vi "Tusk.MessageSenderCore.vi"(5 "Priority?":bool, 7 "Timeout (ms)(-1)":i32=-1, 8 "error in (no error)":errorcluster, 10 "Message":refnum<class "Message.lvclass">, 11 "Tusk in":refnum<class "Tusk.lvclass">) -> (0 "error out":errorcluster, 1 "Timed out?":bool, 3 "Tusk out":refnum<class "Tusk.lvclass">)   [LabVIEW 2018, in "Application.lvlib" / "Tusk.lvclass"]
uses:
  Tusk.lvclass
  Message Class/Message.lvclass
  Tusk.lvclass/Tusk.ctl
  <vilib>/event_ctls.llb/usereventprio.ctl
  Exceptions Class/Exceptions.lvclass
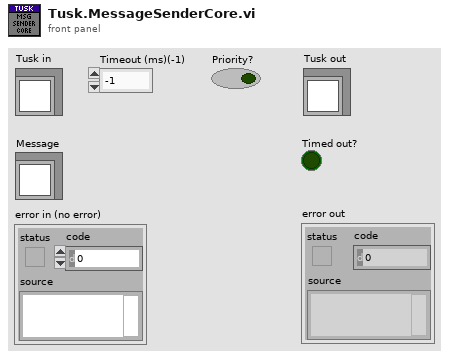
[diagram p1: front panel]
types:
  T1 = typedef "Type.ctl" = enum16{"None", "Queue", "Event", "Notifier"}
  T2 = typedef "usereventprio.ctl" = enum32{"high priority", "normal priority"}
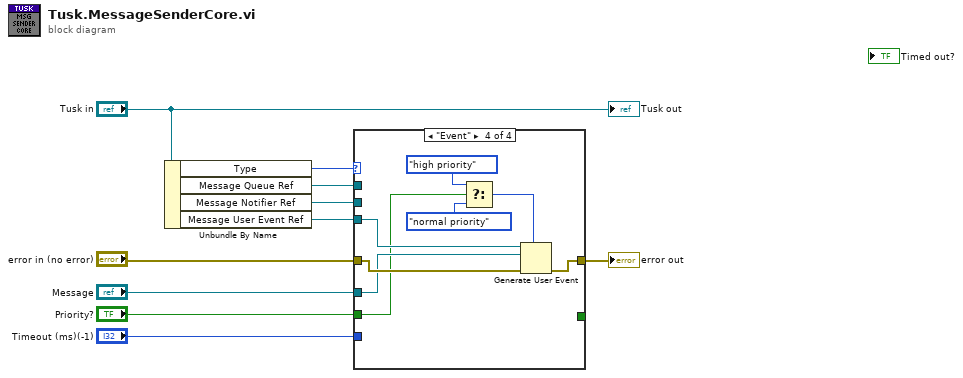
[diagram p0: block diagram]
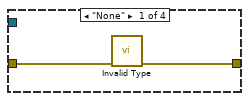
[diagram p2: hidden frame]
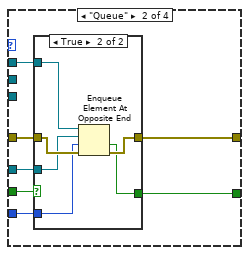
[diagram p3: hidden frame]
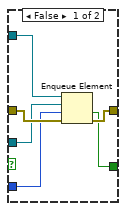
[diagram p4: hidden frame]
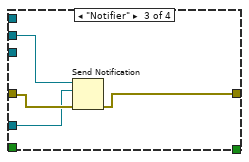
[diagram p5: hidden frame]
diagram:
  n1 = Unbundle By Name("Tusk in") -> ("Type"=w9:T1, "Message Queue Ref"=w8:refnum<queue>, "Message Notifier Ref"=w7:refnum<notifier>, "Message User Event Ref"=w6:refnum<user-event>)
  n2 = case shown="\"Event\"" w9 {
    tunnel: w8 -> [_ w16 _ _]
    tunnel: w7 -> [_ _ w34 _]
    tunnel: w6 -> [_ _ _ w42]
    tunnel: "error in (no error)" -> [w12 w19 w35 w43]
    tunnel: [w11 w14 w32 w40] -> w1
    tunnel: "Priority?" -> [_ w17 _ w36]
    tunnel: "Message" -> [_ w18 w33 w41]
    tunnel: "Timeout (ms)(-1)" -> [_ w15 _ _]
    tunnel: [_ w13 _ _] -> _
    frame "None" {
      n3 = call "Invalid Type.vi"("error in (no error)"=w12) -> ("error out"=w11:errorcluster)  [unwired: 10 in]
    }
    frame "Queue" {
      n4 = case shown="True" w17 {
        tunnel: w19 -> [w24 w31]
        tunnel: w18 -> [w23 w29]
        tunnel: w16 -> [w25 w30]
        tunnel: w15 -> [w22 w28]
        tunnel: [w21 w27] -> w14
        tunnel: [w20 w26] -> w13
        frame False {
          n5 = Enqueue Element(queue=w25, element=w23, timeout in ms (-1)=w22, error in (no error)=w24) -> (timed out?=w20:bool, error out=w21:errorcluster)  [unwired: 1 out]
        }
        frame True {
          n6 = Enqueue Element At Opposite End(queue=w30, element=w29, timeout in ms (-1)=w28, error in (no error)=w31) -> (timed out?=w26:bool, error out=w27:errorcluster)  [unwired: 1 out]
        }
      }
    }
    frame "Notifier" {
      n7 = Send Notification(notification=w33, notifier=w34, error in (no error)=w35) -> (error out=w32:errorcluster)  [unwired: 1 out]
    }
    frame "Event" {
      n8 = Select(t=usereventprio."high priority" ("priority (normal)"), s=w36, f=usereventprio."normal priority" ("priority (normal)")) -> (s? t:f=w39:T2)
      n9 = Generate User Event(priority (normal)=w39, user event=w42, event data cluster=w41, error in=w43) -> (error out=w40:errorcluster)  [unwired: 1 out]
    }
  }
  "error out" <- w1
  "Tusk out" <- "Tusk in"
